vi "AuMT8852B EUT Fail Register Enable.vi"(5 "Flags (all disabled)":T1, 7 "Set/Get (Set)":enum16{"Set", "Get"}(ring), 8 "error in (no error)":errorcluster, 10 "Value (-1)":i32=-1, 11 "VISA session":refnum<visa-resource-name>) -> (0 "error out":errorcluster, 2 "error code":i32, 3 "VISA session out":refnum<visa-resource-name>, 4 "Flags out":T1, 6 "Value out":i32)   [LabVIEW 2017]
doc: "Anritsu MT8852B Bluetooth Tester\n\nIndicates which bits of the Equipment Test Fail Register will cause a Service Request (SRQ). The value can be written as an integer (0-255), or as a cluster of flags.\n\nBit 7 (most significant bit) - Output power test.\nBit 6 - Power control test.\nBit 5 - Initial carrier test.\nBit 4 - Carrier drift test.\nBit 3 - Modulation test.\nBit 2 - Single-slot sensitivity test.\nBit 1 - Multiple-slot sensitivity test.\nBit 0 (least significant bit) - Maximum power test.\n\nINPUTS\nSet/Get - whether the values are being written to or read from the instrument.\nFlags - individual values to assign to the register.\nValue - integer value (0-255) to be written to the register. Leave this input unwired if you are using the Flags input.\n\nOUTPUTS\nFlags out - value of each bit in the register.\nValue out - integer value (0-255) of the register."
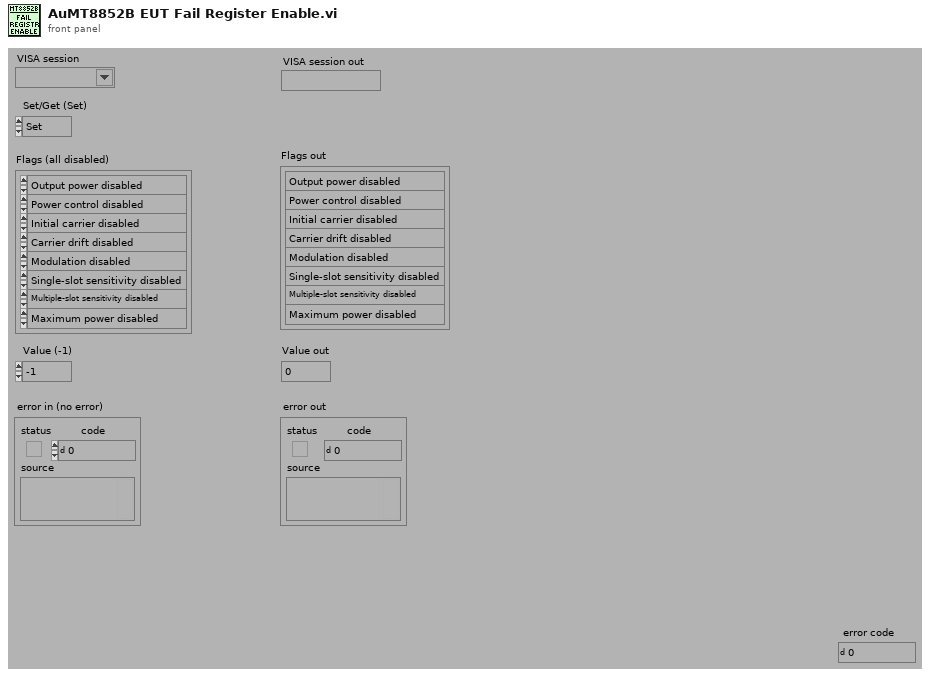
[diagram p1: front panel]
types:
  T1 = cluster{"Output power":enum16{"Output power disabled", "Output power enabled"}, "Power control":enum16{"Power control disabled", "Power control enabled"}, "Initial carrier":enum16{"Initial carrier disabled", "Initial carrier enabled"}, "Carrier drift":enum16{"Carrier drift disabled", "Carrier drift enabled"}, "Modulation":enum16{"Modulation disabled", "Modulation enabled"}, "Single-slot sensitivity":enum16{"Single-slot sensitivity disabled", "Single-slot sensitivity enabled"}, "Multiple-slot sensitivity":enum16{"Multiple-slot sensitivity disabled", "Multiple-slot sensitivity enabled"}, "Maximum power":enum16{"Maximum power disabled", "Maximum power enabled"}}
  T2 = enum16{"Simulate", "Range check", "Cache", "Query instrument status"}
  T3 = cluster{"[0]":i16, "[1]":i16, "[2]":i16, "[3]":i16, "[4]":i16, "[5]":i16, "[6]":i16, "[7]":i16}
  T4 = enum16{"Maximum power disabled", "Maximum power enabled"}
  T5 = enum16{"Multiple-slot sensitivity disabled", "Multiple-slot sensitivity enabled"}
  T6 = enum16{"Single-slot sensitivity disabled", "Single-slot sensitivity enabled"}
  T7 = enum16{"Modulation disabled", "Modulation enabled"}
  T8 = enum16{"Carrier drift disabled", "Carrier drift enabled"}
  T9 = enum16{"Initial carrier disabled", "Initial carrier enabled"}
  T10 = enum16{"Power control disabled", "Power control enabled"}
  T11 = enum16{"Output power disabled", "Output power enabled"}
  T12 = cluster{bool, bool, bool, bool, bool, bool, bool, bool}
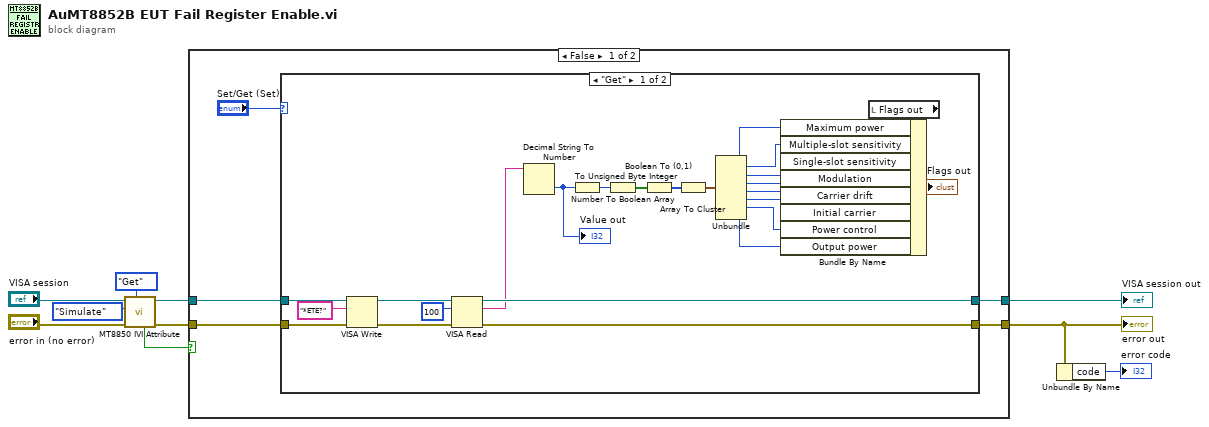
[diagram p0: block diagram]
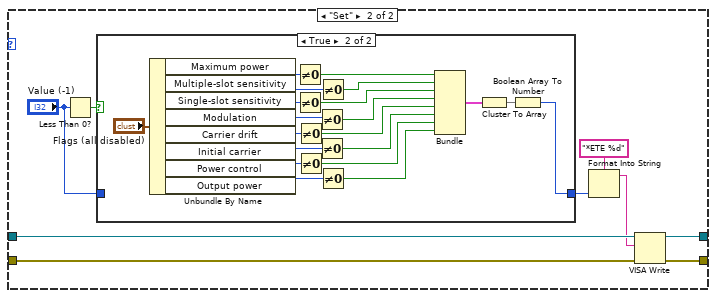
[diagram p2: hidden frame]
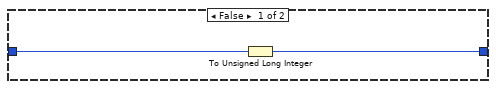
[diagram p3: hidden frame]
diagram:
  n1 = call <instrlib>:"MT8850 IVI Attribute.vi"("Set/Get (Set)"=enum16{"Set", "Get"}."Get", "error in (no error)"="error in (no error)", "Flag (Simulate)"=T2."Simulate", "VISA session"="VISA session") -> ("error out"=w6:errorcluster, "VISA session out"=w7:refnum<visa-resource-name>, "Value out"=w3:bool)  [unwired: 5 in]
  n2 = case shown="False" w3 {
    tunnel: [w12 w71] -> w1
    tunnel: [w13 w72] -> w8
    tunnel: w7 -> [w15 w72]
    tunnel: w6 -> [w14 w71]
    frame False {
      n3 = case shown="\"Get\"" "Set/Get (Set)" {
        tunnel: w15 -> [w39 w48]
        tunnel: w14 -> [w38 w47]
        tunnel: [w34 w44] -> w13
        tunnel: [w33 w43] -> w12
        frame "Get" {
          n4 = VISA Write(VISA resource name=w39, write buffer="*ETE?" ("write buffer (\"\")"), error in (no error)=w38) -> (VISA resource name out=w36:refnum<visa-resource-name>, error out=w35:errorcluster)  [unwired: 1 out]
          n5 = VISA Read(VISA resource name=w36, byte count=u32 100 ("byte count (0)"), error in (no error)=w35) -> (VISA resource name out=w34:refnum<visa-resource-name>, read buffer=w31:string, error out=w33:errorcluster)  [unwired: 1 out]
          n6 = Decimal String To Number(string=w31) -> (number=w26:i32)  [unwired: 2 in, 1 out]
          "Value out" <- w26
          n7 = To Unsigned Byte Integer(number=w26) -> (unsigned 8bit integer=w27:u8)
          n8 = Number To Boolean Array(number=w27) -> (Boolean array=w28:bool[])
          n9 = Boolean To (0,1)(Boolean=w28) -> (0, 1=w29:i16[])
          n10 = Array To Cluster(array=w29) -> (cluster=w30:T3)
          n11 = Unbundle(w30) -> ("[0]"=w17:i16, "[1]"=w19:i16, "[2]"=w21:i16, "[3]"=w23:i16, "[4]"=w22:i16, "[5]"=w20:i16, "[6]"=w18:i16, "[7]"=w16:i16)
          n12 = local read "Flags out"() -> (w25:T1)
          n13 = Bundle By Name(cluster=w25, "Maximum power"=w17, "Multiple-slot sensitivity"=w19, "Single-slot sensitivity"=w21, "Modulation"=w23, "Carrier drift"=w22, "Initial carrier"=w20, "Power control"=w18, "Output power"=w16) -> (→"Flags out":T1)
        }
        frame "Set" {
          n14 = Less Than 0?(x="Value (-1)") -> (x < 0?=w41:bool)
          n15 = case shown="True" w41 {
            tunnel: [w49 w61] -> w45
            tunnel: "Value (-1)" -> [w50 _]
            frame False {
              n16 = To Unsigned Long Integer(number=w50) -> (unsigned 32bit integer=w49:u32)
            }
            frame True {
              n17 = Unbundle By Name("Flags (all disabled)") -> ("Maximum power"=w70:T4, "Multiple-slot sensitivity"=w56:T5, "Single-slot sensitivity"=w55:T6, "Modulation"=w54:T7, "Carrier drift"=w53:T8, "Initial carrier"=w52:T9, "Power control"=w51:T10, "Output power"=w59:T11)
              n18 = Not Equal To 0?(x=w70) -> (x != 0?=w69:bool)
              n19 = Not Equal To 0?(x=w55) -> (x != 0?=w67:bool)
              n20 = Not Equal To 0?(x=w53) -> (x != 0?=w65:bool)
              n21 = Not Equal To 0?(x=w51) -> (x != 0?=w58:bool)
              n22 = Not Equal To 0?(x=w54) -> (x != 0?=w66:bool)
              n23 = Not Equal To 0?(x=w52) -> (x != 0?=w64:bool)
              n24 = Not Equal To 0?(x=w56) -> (x != 0?=w68:bool)
              n25 = Not Equal To 0?(x=w59) -> (x != 0?=w57:bool)
              n26 = Bundle(w69, w68, w67, w66, w65, w64, w58, w57) -> (w63:T12)  [unwired: 1 in]
              n27 = Cluster To Array(cluster=w63) -> (array=w62:bool[])
              n28 = Boolean Array To Number(Boolean array=w62) -> (number=w61:u32)
            }
          }
          n29 = Format Into String(format string="*ETE %d" ("Format String"), w45) -> (resulting string=w42:string)  [unwired: 2 in, 1 out]
          n30 = VISA Write(VISA resource name=w48, write buffer=w42, error in (no error)=w47) -> (VISA resource name out=w44:refnum<visa-resource-name>, error out=w43:errorcluster)  [unwired: 1 out]
        }
      }
    }
    frame True {
    }
  }
  "error out" <- w1
  "VISA session out" <- w8
  n31 = Unbundle By Name(w1) -> ("code"=→"error code":i32)
